vi "GetDiagramOutputs.vi"(6 "error in":errorcluster, 9 "Loop in":refnum<class "Loop.lvclass">) -> (0 "error out":errorcluster, 3 "Loop out":refnum<class "Loop.lvclass">, 4 "output terminals":refnum<class "Terminal.lvclass">[][](array[class]))   [LabVIEW 2014, in "Raspberry Pi Compatible Compiler for LabVIEW.lvlib" / "Loop.lvclass"]
uses:
  Loop.lvclass
  Terminal/Terminal.lvclass
  Loop.lvclass/Loop.ctl
  ShiftRegister/ShiftRegister.lvclass/ShiftRegister.ctl
  Tunnel/Tunnel.lvclass/Tunnel.ctl
  Structure/Structure.lvclass
  ShiftRegister/ShiftRegister.lvclass
  Tunnel/Tunnel.lvclass
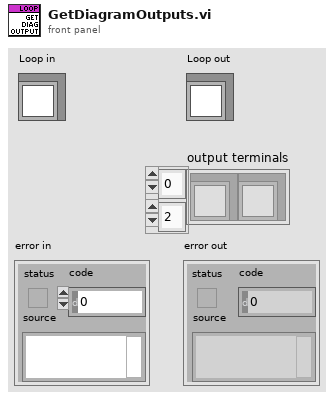
[diagram p1: front panel]
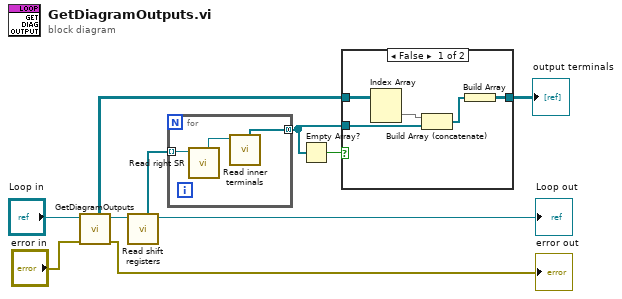
[diagram p0: block diagram]
diagram:
  n1 = call-parent "GetDiagramOutputs.vi"("error in"="error in", "Structure in"="Loop in") -> ("error out"=→"error out":errorcluster, "Structure out"=w8:refnum<class "Loop.lvclass">, "output terminals"=w6:refnum<class "Terminal.lvclass">[][])  [unwired: 5 in]
  n2 = call "Read shift registers.vi"("Loop in"=w8) -> ("Loop out"=→"Loop out":refnum<class "Loop.lvclass">, "shift registers"=w7:refnum<class "ShiftRegister.lvclass">[])  [unwired: 7 in]
  n3 = for {
    tunnel: w7 -> [w13] mode=indexing
    tunnel: [w11] -> w1 mode=concatenating
    n4 = call "Read right SR.vi"("ShiftRegister in"=w13) -> ("right SR"=w12:refnum<class "RightShiftRegister.lvclass">)  [unwired: 7 in, 1 out]
    n5 = call "Read inner terminals.vi"("Tunnel in"=w12) -> ("inner terminals"=w11:refnum<class "Terminal.lvclass">[])  [unwired: 7 in, 1 out]
  }
  n6 = Empty Array?(array=w1) -> (empty?=w2:bool)
  n7 = case shown="False" w2 {
    tunnel: w6 -> [w18 w19]
    tunnel: w1 -> [w16 _]
    tunnel: [w15 w19] -> w3
    frame False {
      n8 = Index Array(array=w18) -> (element=w17:refnum<class "Terminal.lvclass">[])  [unwired: 2 in]
      n9 = Build Array (concatenate)(w17, w16) -> (w14:refnum<class "Terminal.lvclass">[])
      n10 = Build Array(w14) -> (w15:refnum<class "Terminal.lvclass">[][])
    }
    frame True {
    }
  }
  "output terminals" <- w3
